vi "sub-auto size vi fp.vi"(8 "error in (no error)":errorcluster caption="错误输入（无错误）", 9 "btn ref":refnum<vi>, 10 "str ref":refnum<vi>, 11 "vi ref":refnum<vi>) -> (0 "error out":errorcluster caption="错误输出")   [LabVIEW 2011]
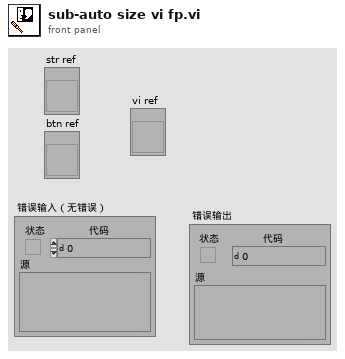
[diagram p1: front panel]
types:
  T1 = typedef "LVRectTypeDef.ctl" = cluster{"left":i16, "top":i16, "right":i16, "bottom":i16}
  T2 = typedef "LVPositionTypeDef.ctl" = cluster{"Left":i32, "Top":i32}
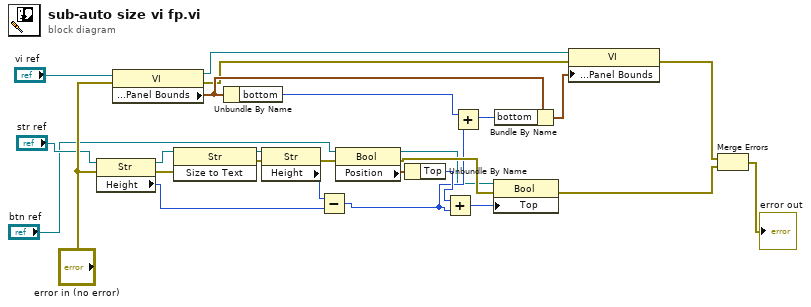
[diagram p0: block diagram]
diagram:
  n1 = property on="属性节点" class="Str"(reference="str ref", error in="error in (no error)") -> (reference out=w2:refnum<vi>, error out=w25:errorcluster, "Height"=w23:u32)
  n2 = property class="VI"(reference="vi ref", error in="error in (no error)") -> (reference out=w9:refnum<vi>, error out=w8:errorcluster, "Front Panel Window:Panel Bounds"=w15:T1)
  n3 = invoke on="调用节点" class="Str" method="Size to Text"(reference=w2, error in=w25) -> (reference out=w11:refnum<vi>, error out=w26:errorcluster)  [unwired: 1 in, 1 out]
  n4 = Unbundle By Name(w15) -> ("bottom"=w17:i16)
  n5 = property on="属性节点" class="Str"(reference=w11, error in=w26) -> (error out=w22:errorcluster, "Height"=w24:u32)  [unwired: 1 out]
  n6 = Subtract(x=w24, y=w23) -> (x-y=w16:u32)
  n7 = property on="属性节点" class="Bool"(reference="btn ref", error in=w22) -> (reference out=w10:refnum<vi>, error out=w18:errorcluster, "Position"=w21:T2)
  n8 = Unbundle By Name(w21) -> ("Top"=w20:i32)
  n9 = Add(x=w20, y=w16) -> (x+y=w19:u32)
  n10 = Add(x=w17, y=w16) -> (x+y=w14:u32)
  n11 = property on="属性节点" class="Bool"(reference=w10, error in=w18, "Top"=w19) -> (error out=w5:errorcluster)  [unwired: 1 out]
  n12 = Bundle By Name(cluster=w15, "bottom"=w14) -> (w13:T1)
  n13 = property class="VI"(reference=w9, error in=w8, "Front Panel Window:Panel Bounds"=w13) -> (error out=w6:errorcluster)  [unwired: 1 out]
  n14 = Merge Errors(w6, w5) -> (→"error out":errorcluster)
